vi "Set message.vi"(10 "WampMessage MsgPack":refnum<class "WampMessage MsgPack.lvclass">, 11 "IHandleUnsubscribed MsgPack in":refnum<class "IHandleUnsubscribed MsgPack.lvclass">) -> (3 "IHandleUnsubscribed MsgPack out":refnum<class "IHandleUnsubscribed MsgPack.lvclass">)   [LabVIEW 2020, in "wamplv.lvlib" / "IHandleUnsubscribed MsgPack.lvclass"]
uses:
  IHandleUnsubscribed MsgPack.lvclass
  IHandleUnsubscribed MsgPack.lvclass/IHandleUnsubscribed MsgPack.ctl
  SerialisedMessages/MsgPackMessage/WampMessage MsgPack.lvclass
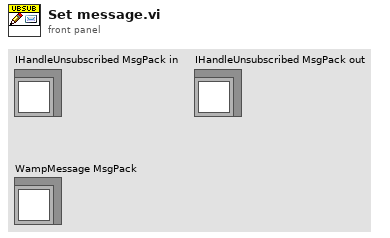
[diagram p1: front panel]
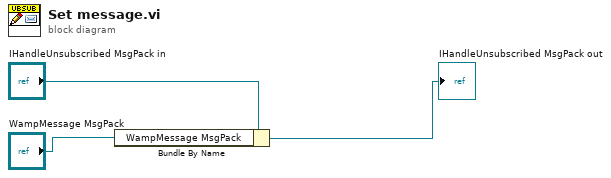
[diagram p0: block diagram]
diagram:
  n1 = Bundle By Name(cluster="IHandleUnsubscribed MsgPack in", "WampMessage MsgPack"="WampMessage MsgPack") -> (→"IHandleUnsubscribed MsgPack out":refnum<class "IHandleUnsubscribed MsgPack.lvclass">)
